vi "main - Copy.vi"() -> ()   [LabVIEW 2016]
panel:
  out "flag":bool
  out "index":dbl
  out "z":dbl
  out "y":dbl
  out "x":dbl
  in  "stop":bool
  out "1":string
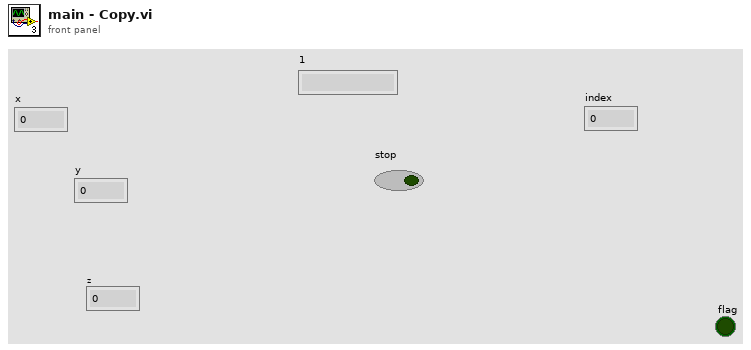
[diagram p1: front panel]
types:
  T1 = enum16{"1", "volume_+", "volume_-", "frequency+", "frequency-", "note1_selec", "note2_selec", "idle 2", "idle 3"}
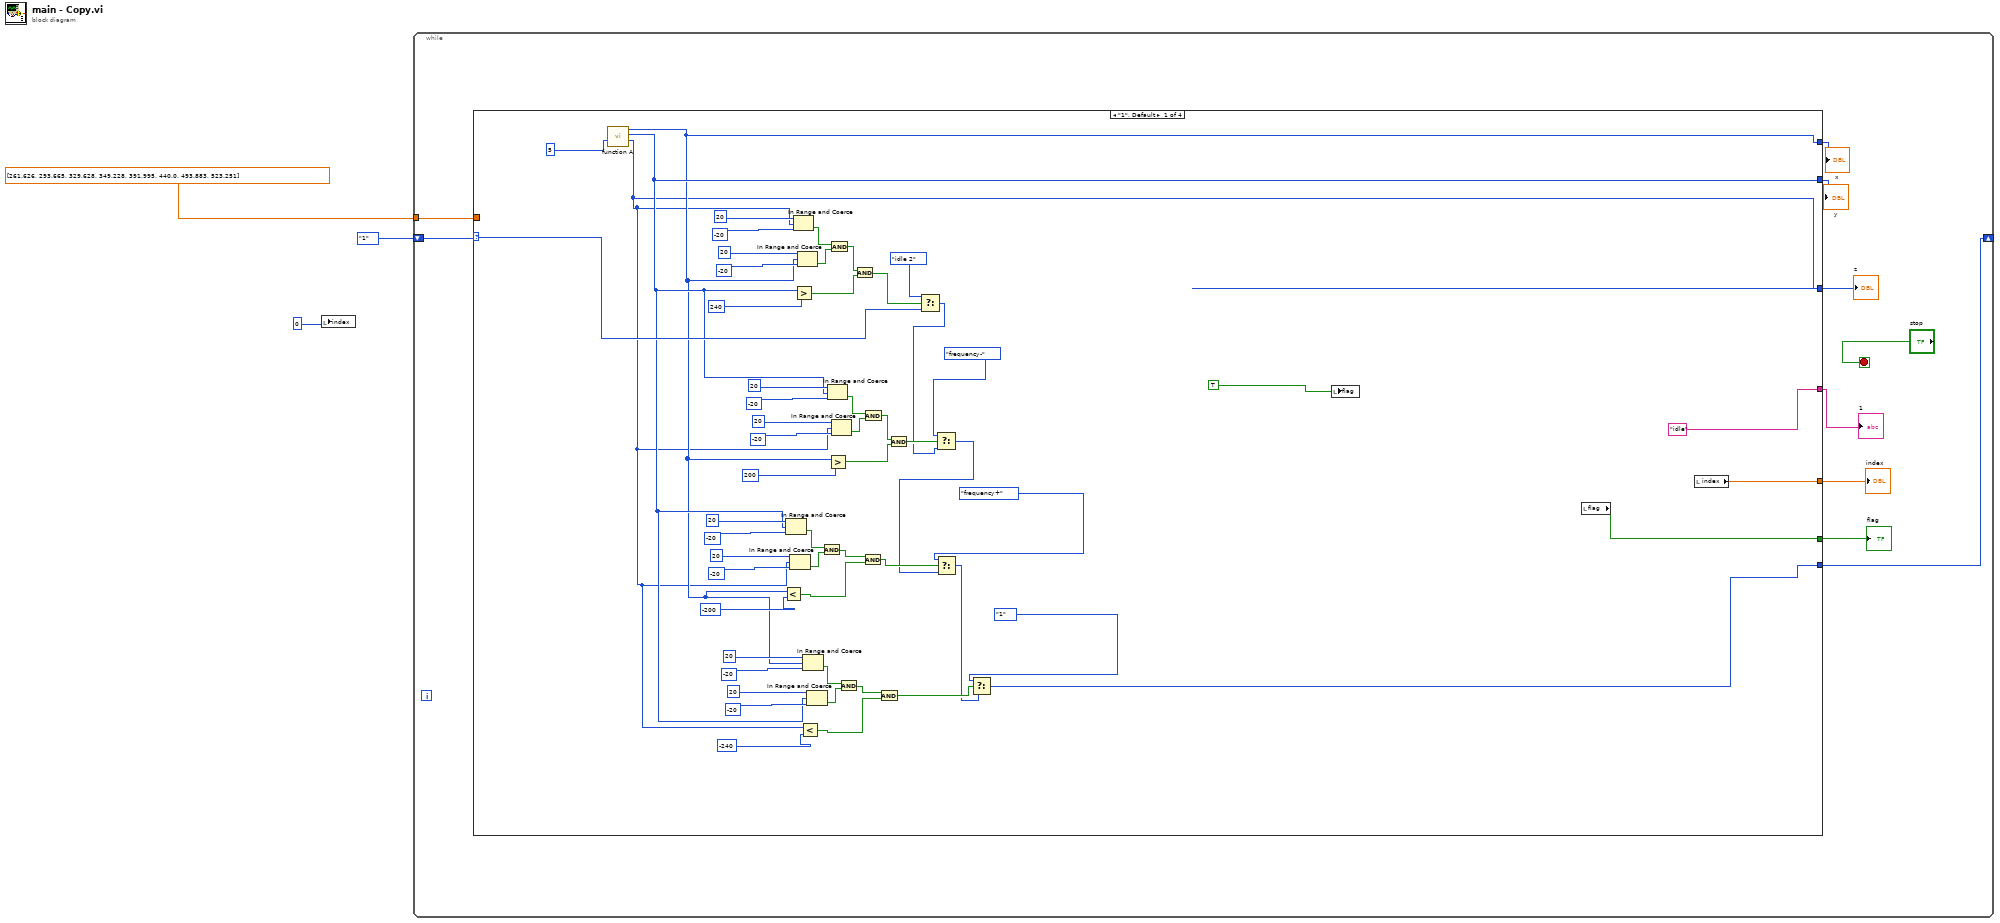
[diagram p0: block diagram]
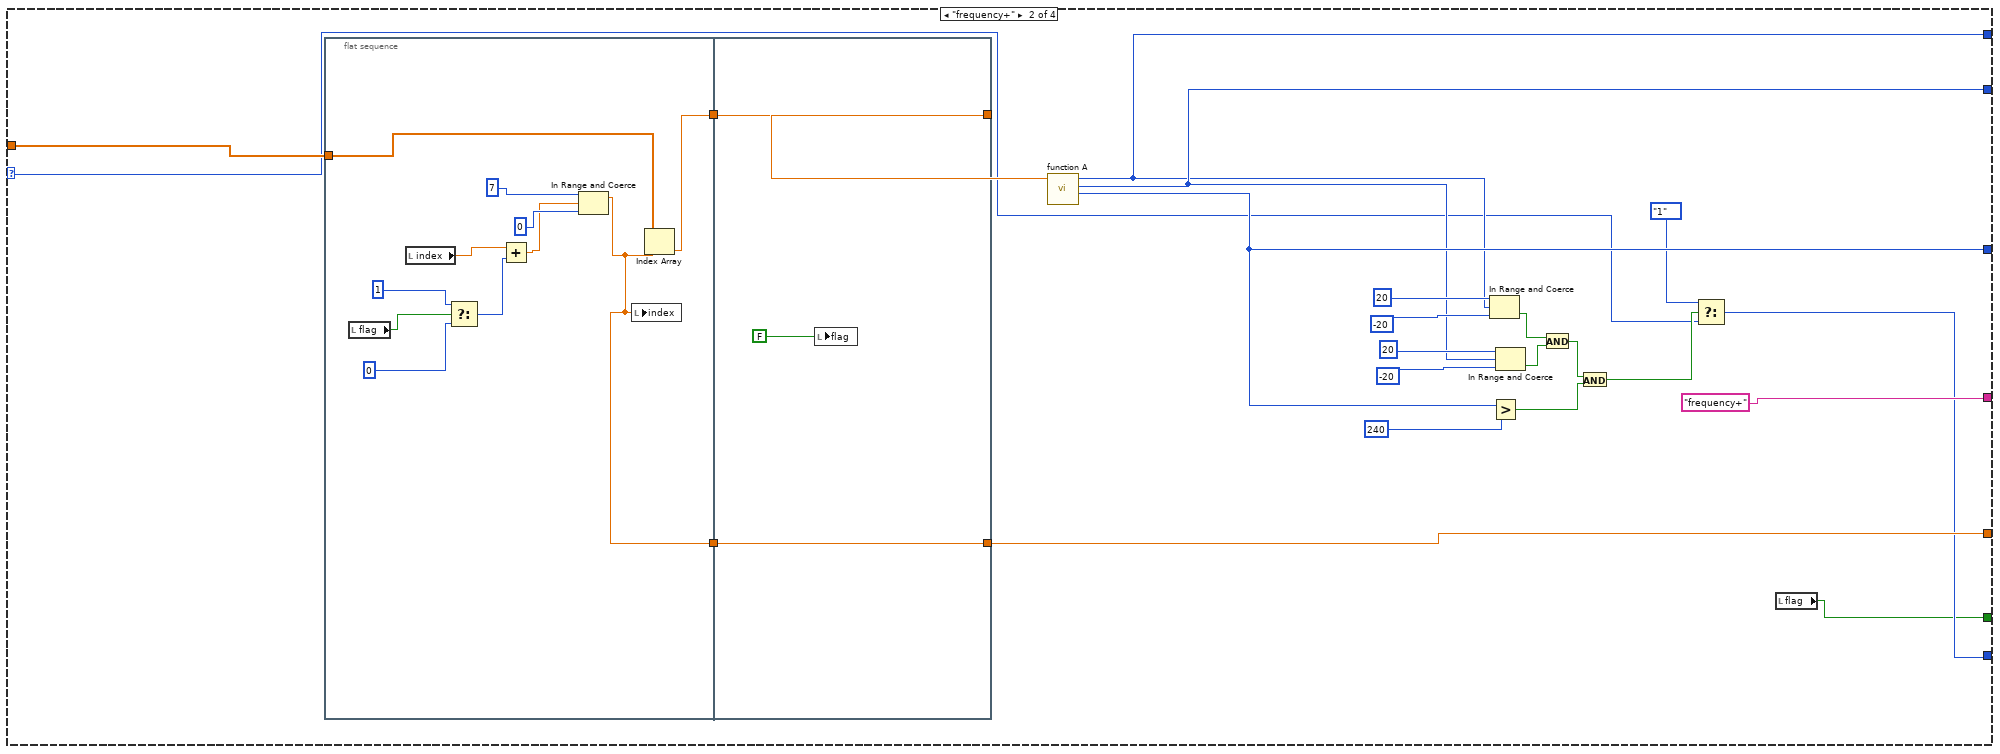
[diagram p2: hidden frame]
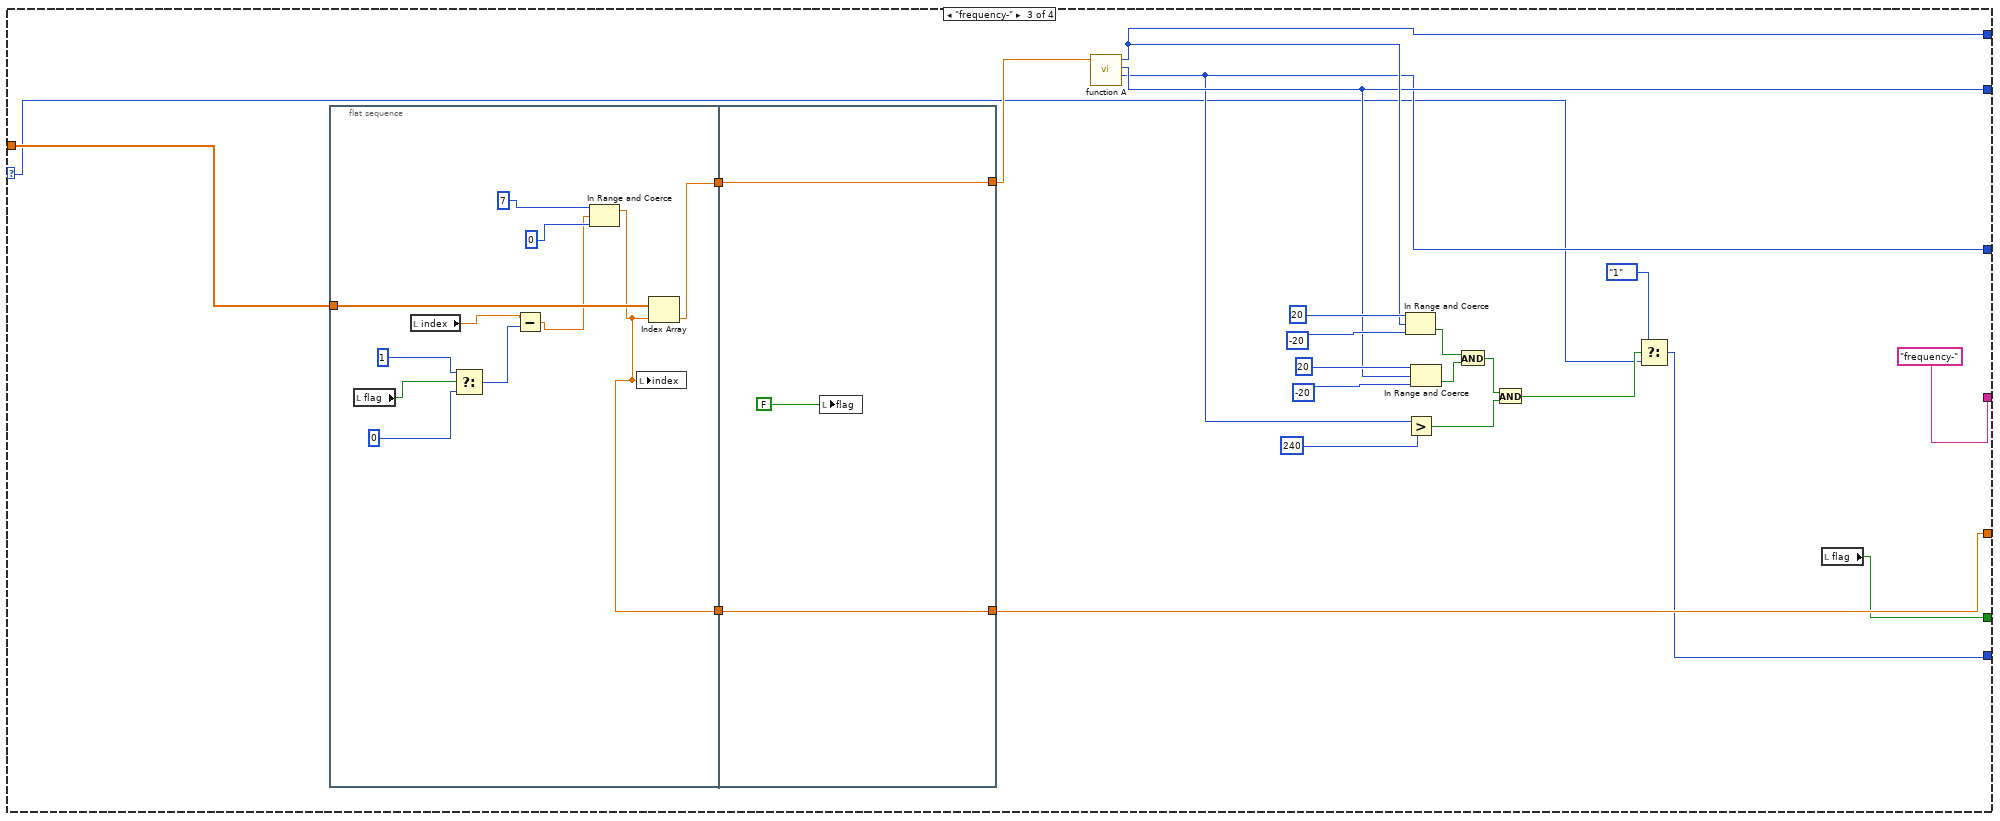
[diagram p3: hidden frame]
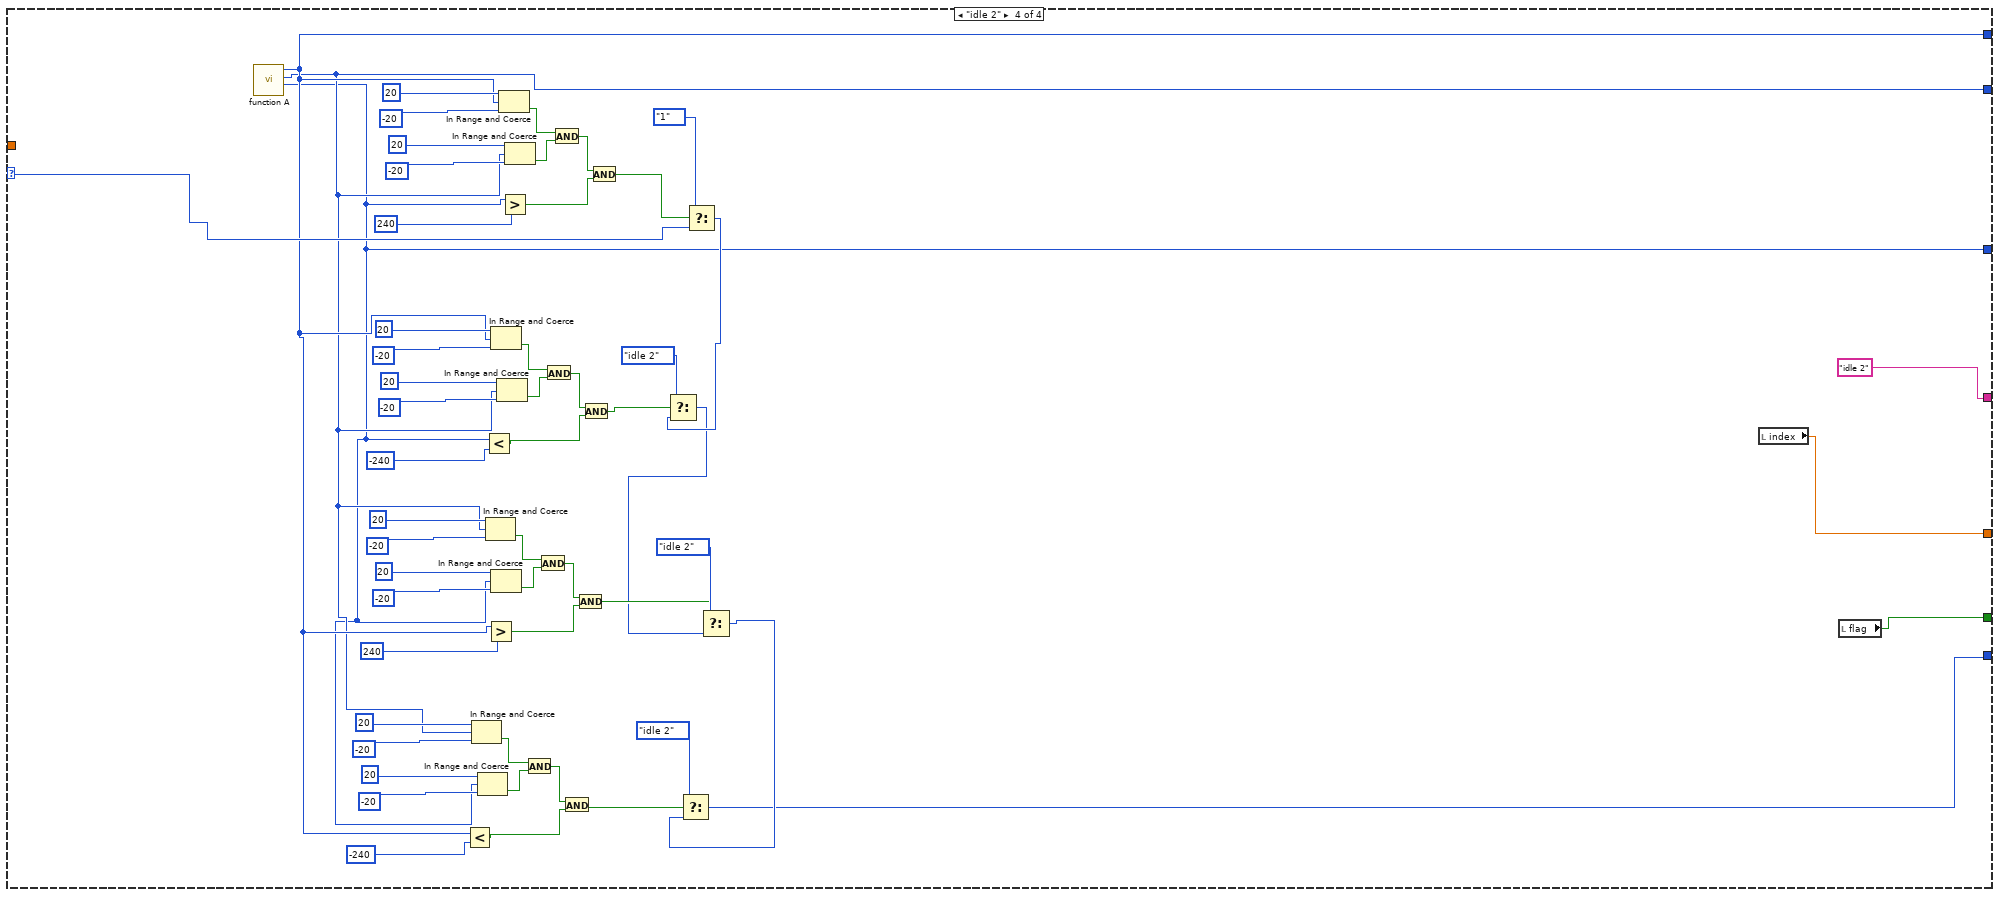
[diagram p4: hidden frame]
diagram:
  n1 = local write "index"(0) -> ()
  n2 = while {
    shift-right: [w7] -> _
    shift-left: T1."1" -> [w8]
    tunnel: dbl[] [261.626, 293.665, 329.628, 349.228, 391.995, 440.0, 493.883, 523.251] -> [w6]
    stop <- "stop" stop-if-true
    n3 = case shown="\"1\", Default" w8 {
      selector: w8 -> [w59 w74 w111 w189]
      tunnel: ["idle" "frequency+" "frequency-" "idle 2"] -> w13
      tunnel: [w16 w76 w115 w149] -> w11
      tunnel: [w19 w77 w114 w148] -> w10
      tunnel: [w15 w78 w113 w147] -> w9
      tunnel: [w22 w72 w109 w151] -> w7
      tunnel: w6 -> [_ w91 w127 _]
      tunnel: [w18 w90 w125 w146] -> w5
      tunnel: [w20 w71 w108 w150] -> w4
      frame "1", Default {
        n4 = call "function A.vi"("volume"=5) -> ("AccelerationZ"=w15:i16, "AccelerationY"=w19:i16, "AccelerationX"=w16:i16)  [unwired: 8 in]
        n5 = Less?(x=w16, y=-200) -> (x < y?=w41:bool)
        n6 = In Range and Coerce(upper limit=20, x=w19, lower limit=-20) -> (In Range?=w44:bool)  [unwired: 1 out]
        n7 = In Range and Coerce(upper limit=20, x=w15, lower limit=-20) -> (In Range?=w43:bool)  [unwired: 1 out]
        n8 = In Range and Coerce(upper limit=20, x=w15, lower limit=-20) -> (In Range?=w64:bool)  [unwired: 1 out]
        n9 = Greater?(x=w19, y=240) -> (0:w61:bool)
        n10 = In Range and Coerce(upper limit=20, x=w16, lower limit=-20) -> (In Range?=w63:bool)  [unwired: 1 out]
        n11 = Less?(x=w15, y=-240) -> (x < y?=w27:bool)
        n12 = In Range and Coerce(upper limit=20, x=w16, lower limit=-20) -> (In Range?=w30:bool)  [unwired: 1 out]
        n13 = In Range and Coerce(upper limit=20, x=w19, lower limit=-20) -> (In Range?=w29:bool)  [unwired: 1 out]
        n14 = And(x=w44, y=w43) -> (x .and. y?=w42:bool)
        n15 = In Range and Coerce(upper limit=20, x=w19, lower limit=-20) -> (In Range?=w54:bool)  [unwired: 1 out]
        n16 = Greater?(x=w16, y=200) -> (0:w51:bool)
        n17 = And(x=w64, y=w63) -> (x .and. y?=w62:bool)
        n18 = In Range and Coerce(upper limit=20, x=w15, lower limit=-20) -> (In Range?=w53:bool)  [unwired: 1 out]
        n19 = And(x=w30, y=w29) -> (x .and. y?=w28:bool)
        n20 = And(x=w62, y=w61) -> (x .and. y?=w60:bool)
        n21 = And(x=w42, y=w41) -> (x .and. y?=w39:bool)
        n22 = And(x=w54, y=w53) -> (x .and. y?=w52:bool)
        n23 = And(x=w28, y=w27) -> (x .and. y?=w24:bool)
        n24 = And(x=w52, y=w51) -> (x .and. y?=w50:bool)
        n25 = Select(t=T1."idle 2", s=w60, f=w59) -> (s? t:f=w49:T1)
        n26 = Select(t=T1."frequency-", s=w50, f=w49) -> (s? t:f=w38:T1)
        n27 = Select(t=T1."frequency+", s=w39, f=w38) -> (s? t:f=w23:T1)
        n28 = Select(t=T1."1", s=w24, f=w23) -> (s? t:f=w22:T1)
        n29 = local write "flag"(TRUE) -> ()
        n30 = local read "flag"() -> (w20:bool)
        n31 = local read "index"() -> (w18:dbl)
      }
      frame "frequency+" {
        n32 = flat-sequence {
          tunnel: w91 -> [w103]
          tunnel: [w104] -> w89
          tunnel: [w94] -> w88
          tunnel: [w106] -> w90
          tunnel: [w107] -> w92
          tunnel: w89 -> [w107]
          tunnel: w88 -> [w106]
          frame #0 {
            n33 = local read "flag"() -> (w98:bool)
            n34 = local read "index"() -> (w102:dbl)
            n35 = Select(t=1, s=w98, f=0) -> (s? t:f=w99:i32)
            n36 = Add(x=w102, y=w99) -> (x+y=w95:dbl)
            n37 = In Range and Coerce(upper limit=7, x=w95, lower limit=0) -> (coerced(x)=w94:dbl)  [unwired: 1 out]
            n38 = local write "index"(w94) -> ()
            n39 = Index Array(array=w103, index=w94) -> (element=w104:dbl)
          }
          frame #1 {
            n40 = local write "flag"(FALSE) -> ()
          }
        }
        n41 = call "function A.vi"("frequency 1"=w92) -> ("AccelerationZ"=w78:i16, "AccelerationY"=w77:i16, "AccelerationX"=w76:i16)  [unwired: 8 in]
        n42 = In Range and Coerce(upper limit=20, x=w76, lower limit=-20) -> (In Range?=w82:bool)  [unwired: 1 out]
        n43 = Greater?(x=w78, y=240) -> (0:w79:bool)
        n44 = In Range and Coerce(upper limit=20, x=w77, lower limit=-20) -> (In Range?=w81:bool)  [unwired: 1 out]
        n45 = And(x=w82, y=w81) -> (x .and. y?=w80:bool)
        n46 = And(x=w80, y=w79) -> (x .and. y?=w75:bool)
        n47 = Select(t=T1."1", s=w75, f=w74) -> (s? t:f=w72:T1)
        n48 = local read "flag"() -> (w71:bool)
      }
      frame "frequency-" {
        n49 = flat-sequence {
          tunnel: [w141] -> w129
          tunnel: [w131] -> w128
          tunnel: w127 -> [w137]
          tunnel: [w143] -> w125
          tunnel: [w144] -> w126
          tunnel: w129 -> [w144]
          tunnel: w128 -> [w143]
          frame #0 {
            n50 = local read "flag"() -> (w138:bool)
            n51 = local read "index"() -> (w136:dbl)
            n52 = Select(t=1, s=w138, f=0) -> (s? t:f=w135:i32)
            n53 = Subtract(x=w136, y=w135) -> (x-y=w132:dbl)
            n54 = In Range and Coerce(upper limit=7, x=w132, lower limit=0) -> (coerced(x)=w131:dbl)  [unwired: 1 out]
            n55 = local write "index"(w131) -> ()
            n56 = Index Array(array=w137, index=w131) -> (element=w141:dbl)
          }
          frame #1 {
            n57 = local write "flag"(FALSE) -> ()
          }
        }
        n58 = call "function A.vi"("frequency 1"=w126) -> ("AccelerationZ"=w113:i16, "AccelerationY"=w114:i16, "AccelerationX"=w115:i16)  [unwired: 8 in]
        n59 = In Range and Coerce(upper limit=20, x=w115, lower limit=-20) -> (In Range?=w119:bool)  [unwired: 1 out]
        n60 = Greater?(x=w113, y=240) -> (0:w116:bool)
        n61 = In Range and Coerce(upper limit=20, x=w114, lower limit=-20) -> (In Range?=w118:bool)  [unwired: 1 out]
        n62 = And(x=w119, y=w118) -> (x .and. y?=w117:bool)
        n63 = And(x=w117, y=w116) -> (x .and. y?=w112:bool)
        n64 = Select(t=T1."1", s=w112, f=w111) -> (s? t:f=w109:T1)
        n65 = local read "flag"() -> (w108:bool)
      }
      frame "idle 2" {
        n66 = call "function A.vi"() -> ("AccelerationZ"=w147:i16, "AccelerationY"=w148:i16, "AccelerationX"=w149:i16)  [unwired: 9 in]
        n67 = Less?(x=w149, y=-240) -> (x < y?=w156:bool)
        n68 = In Range and Coerce(upper limit=20, x=w148, lower limit=-20) -> (In Range?=w159:bool)  [unwired: 1 out]
        n69 = In Range and Coerce(upper limit=20, x=w147, lower limit=-20) -> (In Range?=w158:bool)  [unwired: 1 out]
        n70 = Less?(x=w147, y=-240) -> (x < y?=w180:bool)
        n71 = In Range and Coerce(upper limit=20, x=w148, lower limit=-20) -> (In Range?=w170:bool)  [unwired: 1 out]
        n72 = Greater?(x=w149, y=240) -> (0:w167:bool)
        n73 = In Range and Coerce(upper limit=20, x=w149, lower limit=-20) -> (In Range?=w183:bool)  [unwired: 1 out]
        n74 = In Range and Coerce(upper limit=20, x=w147, lower limit=-20) -> (In Range?=w169:bool)  [unwired: 1 out]
        n75 = In Range and Coerce(upper limit=20, x=w148, lower limit=-20) -> (In Range?=w182:bool)  [unwired: 1 out]
        n76 = In Range and Coerce(upper limit=20, x=w149, lower limit=-20) -> (In Range?=w194:bool)  [unwired: 1 out]
        n77 = Greater?(x=w147, y=240) -> (0:w191:bool)
        n78 = In Range and Coerce(upper limit=20, x=w148, lower limit=-20) -> (In Range?=w193:bool)  [unwired: 1 out]
        n79 = And(x=w159, y=w158) -> (x .and. y?=w157:bool)
        n80 = And(x=w170, y=w169) -> (x .and. y?=w168:bool)
        n81 = And(x=w183, y=w182) -> (x .and. y?=w181:bool)
        n82 = And(x=w194, y=w193) -> (x .and. y?=w192:bool)
        n83 = And(x=w157, y=w156) -> (x .and. y?=w153:bool)
        n84 = And(x=w168, y=w167) -> (x .and. y?=w165:bool)
        n85 = And(x=w181, y=w180) -> (x .and. y?=w177:bool)
        n86 = And(x=w192, y=w191) -> (x .and. y?=w190:bool)
        n87 = Select(t=T1."1", s=w190, f=w189) -> (s? t:f=w176:T1)
        n88 = Select(t=T1."idle 2", s=w177, f=w176) -> (s? t:f=w164:T1)
        n89 = Select(t=T1."idle 2", s=w165, f=w164) -> (s? t:f=w152:T1)
        n90 = Select(t=T1."idle 2", s=w153, f=w152) -> (s? t:f=w151:T1)
        n91 = local read "index"() -> (w146:dbl)
        n92 = local read "flag"() -> (w150:bool)
      }
    }
    "1" <- w13
    "x" <- w11
    "y" <- w10
    "z" <- w9
    "index" <- w5
    "flag" <- w4
  }
